vi "HoloLink_get_all_trajectories.vi"(8 "error in (no error)":errorcluster, 11 "session in":refnum<k35>) -> (0 "error out":errorcluster, 2 "AllTrajectories":dbl[][](array[numeric]), 3 "Refnum out":refnum<k35>)   [LabVIEW 2023, in "holoTracker.lvlib"]
uses:
  holoTracker.lvlib
panel:
  # "wavelenght, optical_index, image_size_X, image_size_Y, pixel_size, magnification = holo_info\n\n    propag_param, focus_param, binarisation_param, CCL_param = analyse_parameters\n    distance_ini, nb_plane, propag_step, filter = propag_param\n    high_pass_filter, low_pass_filter = filter\n    #focus parameters unpacking\n    focus_type, sum_size = focus_param\n    #binarisation parameters unpacking\n    nbStdVarThreshold, threshold_target = binarisation_param\n    #CCL parameters unpacking\n    n_connectivity, min_voxel, max_voxel = CCL_param"
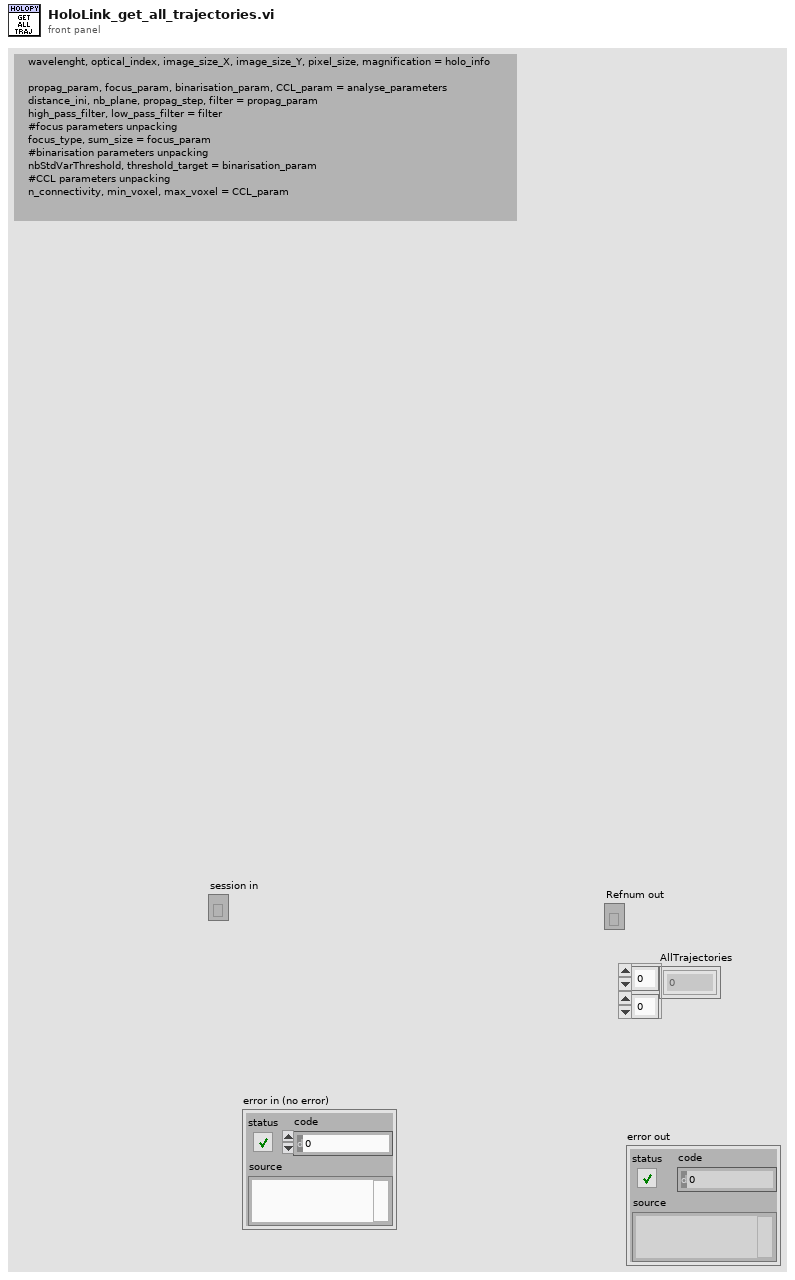
[diagram p1: front panel]
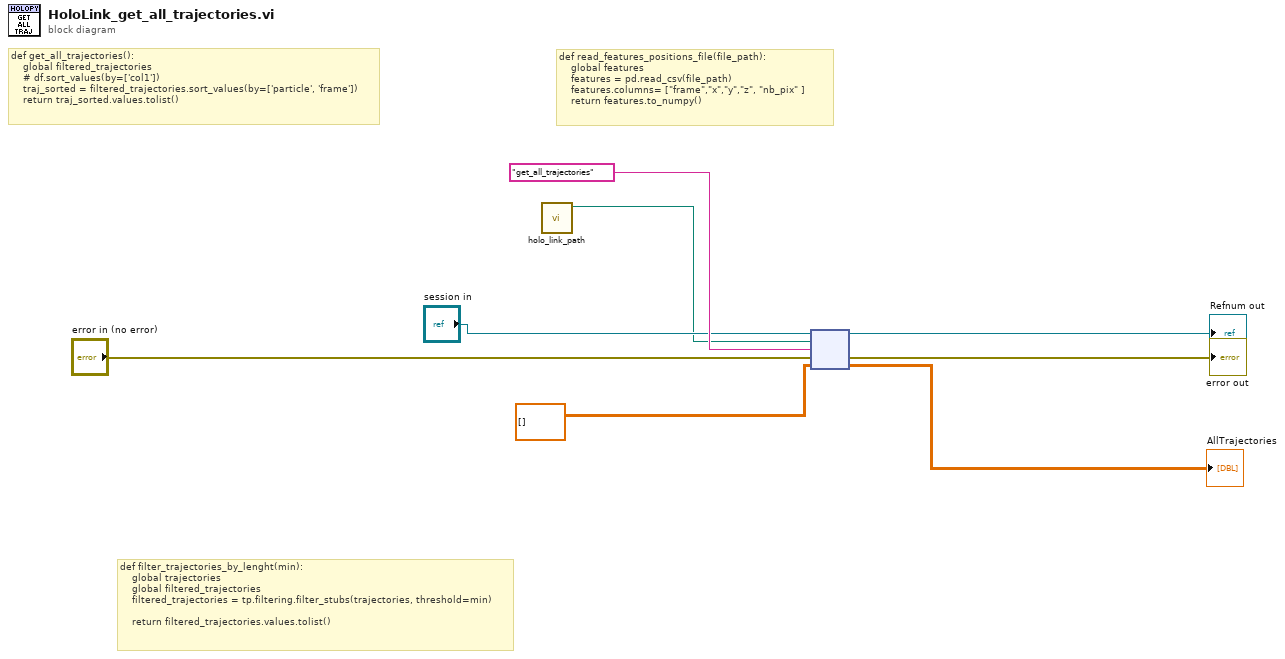
[diagram p0: block diagram]
diagram:
  # "def get_all_trajectories():\n    global filtered_trajectories\n    # df.sort_values(by=['col1'])\n    traj_sorted = filtered_trajectories.sort_values(by=['particle', 'frame'])\n    return traj_sorted.values.tolist()"
  # "def filter_trajectories_by_lenght(min):\n    global trajectories\n    global filtered_trajectories    \n    filtered_trajectories = tp.filtering.filter_stubs(trajectories, threshold=min)\n\n    return filtered_trajectories.values.tolist()"
  # "def read_features_positions_file(file_path):\n    global features\n    features = pd.read_csv(file_path)\n    features.columns= [\"frame\",\"x\",\"y\",\"z\", \"nb_pix\" ]\n    return features.to_numpy()"
  n1 = call "holo_link_path.vi"() -> ("appended path"=w5:path)  [unwired: 11 in]
  n2 = node("session in", w5, "get_all_trajectories" ("function name"), "error in (no error)", dbl[][] []) -> (→"Refnum out":refnum<k35>, →"error out":errorcluster, →"AllTrajectories":dbl[][])  [unwired: 2 out]
